vi "delete channel from configuration.vi"(8 "error in":errorcluster, 10 "TBM channel in":refnum<class "TBM channel.lvclass">, 11 "Shared Library Module configuration in":refnum<class "Shared Library Module configuration.lvclass">) -> (0 "error out":errorcluster, 3 "Shared Library Module configuration out":refnum<class "Shared Library Module configuration.lvclass">)   [LabVIEW 2013, in "Shared Library Module configuration.lvclass"]
doc: "Platypus Framework 1.0.1.60\nNI Systems Engineering - National Instruments"
uses:
  Shared Library Module configuration.lvclass
  <vilib>/NI/Tag Bus Module Framework/channel/TBM channel.lvclass
  <vilib>/NI/Tag Bus/tag/tag descriptor.lvclass/tag descriptor.ctl
  Shared Library Module configuration.lvclass/Shared Library Module configuration.ctl
  <vilib>/NI/Tag Bus/tag/tag descriptor.lvclass
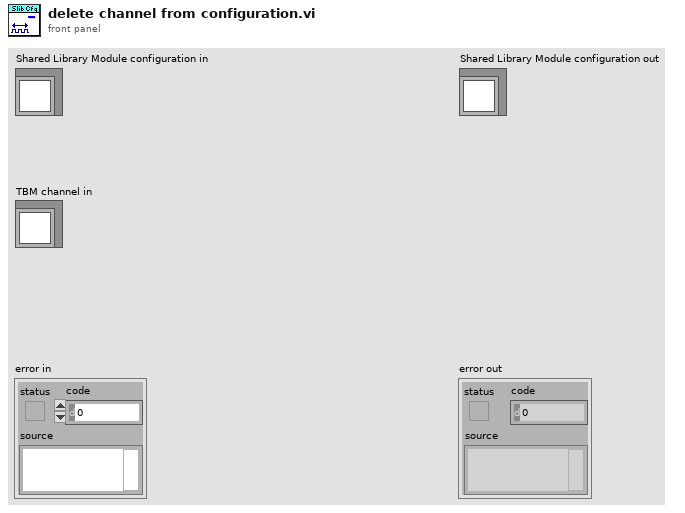
[diagram p1: front panel]
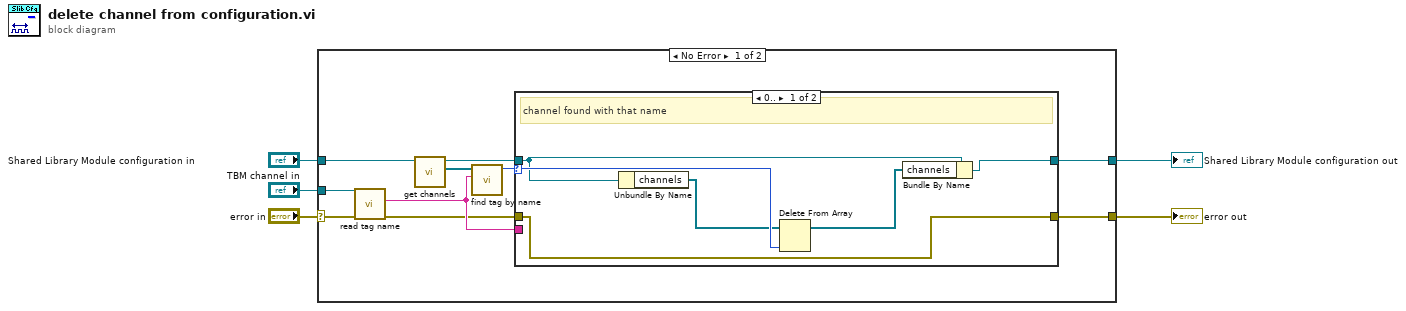
[diagram p0: block diagram]
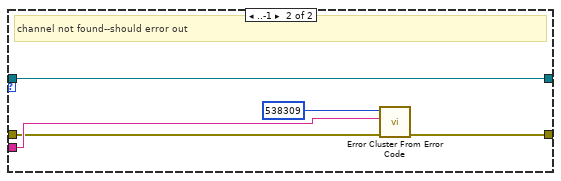
[diagram p2: hidden frame]
diagram:
  n1 = case shown="No Error" "error in" {
    selector: "error in" -> [w8 w27]
    tunnel: "TBM channel in" -> [w14 _]
    tunnel: [w13 w27] -> w4
    tunnel: [w12 w28] -> w3
    tunnel: "Shared Library Module configuration in" -> [w11 w28]
    frame No Error {
      n2 = call <vilib>:"read tag name.vi"("error in"=w8, "system tag in"=w14) -> ("error out"=w6:errorcluster, "name"=w7:string)  [unwired: 7 in, 1 out]
      n3 = call-dynamic "get channels.vi"("Shared Library Module configuration in"=w11) -> ("channels"=w10:refnum<class "TBM channel.lvclass">[], "Shared Library Module configuration out"=w15:refnum<class "Shared Library Module configuration.lvclass">)  [unwired: 9 in]
      n4 = call <vilib>:"find tag by name.vi"("name"=w7, "tags in"=w10) -> ("index"=w9:i32)  [unwired: 9 in]
      n5 = case shown="0.." w9 {
        selector: w9 -> [w21 _]
        tunnel: [w20 w26] -> w13
        tunnel: w7 -> [_ w24]
        tunnel: w6 -> [w20 w23]
        tunnel: w15 -> [w19 w22]
        tunnel: [w16 w22] -> w12
        frame 0.. {
          # "channel found with that name"
          n6 = Unbundle By Name(w19) -> ("channels"=w18:refnum<class "TBM channel.lvclass">[])
          n7 = Delete From Array(array=w18, index=w21) -> (array with subset deleted=w17:refnum<class "TBM channel.lvclass">[])  [unwired: 1 in, 1 out]
          n8 = Bundle By Name(cluster=w19, "channels"=w17) -> (w16:refnum<class "Shared Library Module configuration.lvclass">)
        }
        frame ..-1 {
          # "channel not found--should error out"
          n9 = call <vilib>:"Error Cluster From Error Code.vi"("error in (no error)"=w23, "error message (\"\")"=w24, "error code (0)"=538309) -> ("error out"=w26:errorcluster)  [unwired: 6 in]
        }
      }
    }
    frame Error {
    }
  }
  "error out" <- w4
  "Shared Library Module configuration out" <- w3
